vi "SendMessage.vi"(5 "atributes":variant, 6 "timeout in ms (-1)":i32=-1, 7 "urgent? (F)":bool, 8 "error in":errorcluster, 9 "data":variant, 10 "name":string, 11 "message ref in":refnum<class "CLM_LocalMessage.lvclass">) -> (0 "error out":errorcluster, 3 "message ref out":refnum<class "CLM_LocalMessage.lvclass">, 4 "timed out?":bool)   [LabVIEW 2013, in "CLM_LocalMessage.lvclass"]
uses:
  CLM_LocalMessage.lvclass
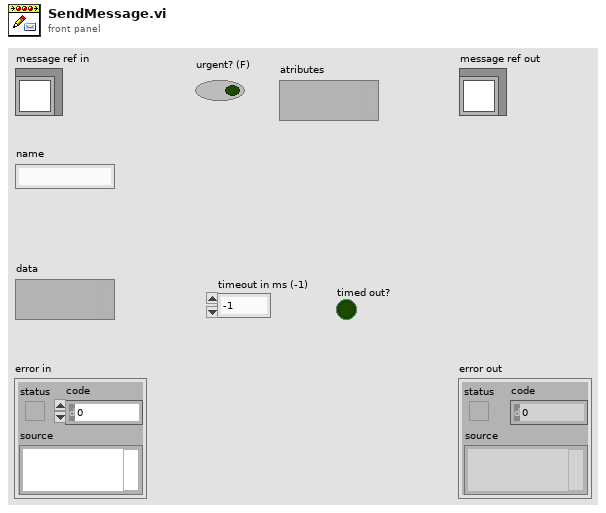
[diagram p1: front panel]
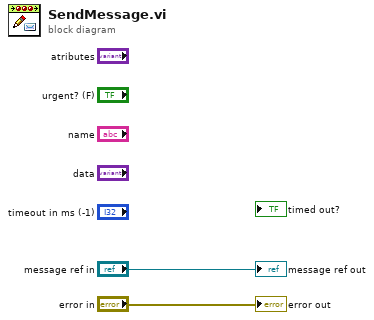
[diagram p0: block diagram]
diagram:
  "error out" <- "error in"
  "message ref out" <- "message ref in"
